vi "SNAKE AND LADDER 2 players final.vi"() -> ()   [LabVIEW 2018]
panel:
  out "dice 2":dbl(ring)
  out "dice 1":dbl(ring)
  out "WINNER":string
  out "Player 2":string
  out "PLAYER 2 LAST VALUE":dbl
  out "PLAYER 2":dbl
  out "PLAYER 2\nNEW VALUE":dbl
  out "NO.OF ROLLS":dbl
  out "PLAYER 1\nNEW VALUE":dbl
  out "PLAYER 1":dbl
  out "PLAYER 1 LAST VALUE":dbl
  out "Player 1":string
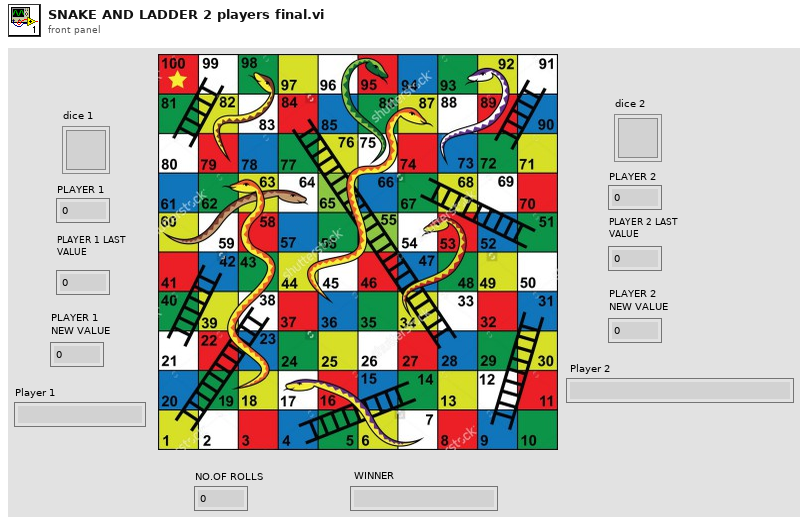
[diagram p1: front panel]
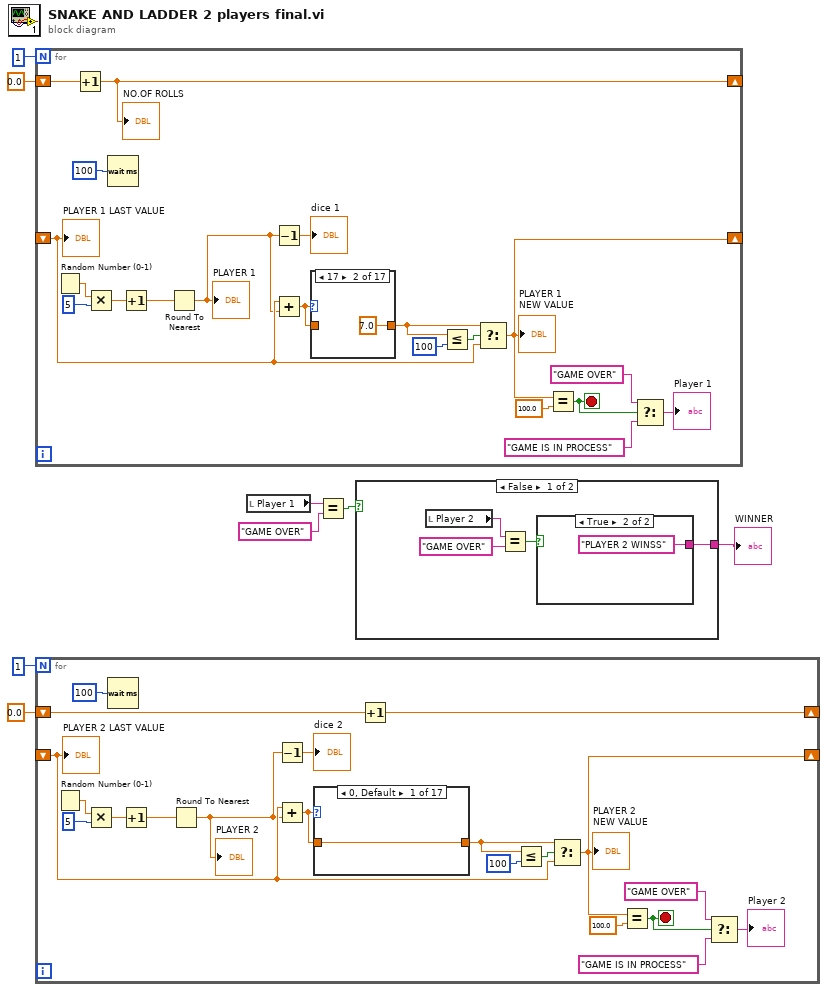
[diagram p0: block diagram]
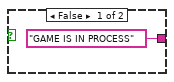
[diagram p2: hidden frame]
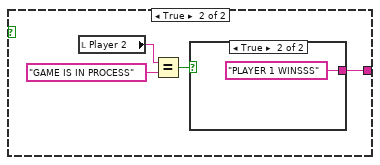
[diagram p3: hidden frame]
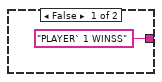
[diagram p4: hidden frame]
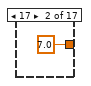
[diagram p5: hidden frame]
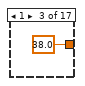
[diagram p6: hidden frame]
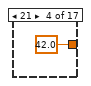
[diagram p7: hidden frame]
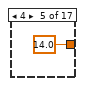
[diagram p8: hidden frame]
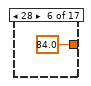
[diagram p9: hidden frame]
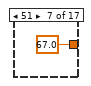
[diagram p10: hidden frame]
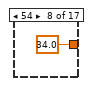
[diagram p11: hidden frame]
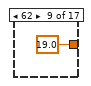
[diagram p12: hidden frame]
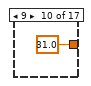
[diagram p13: hidden frame]
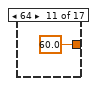
[diagram p14: hidden frame]
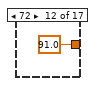
[diagram p15: hidden frame]
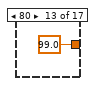
[diagram p16: hidden frame]
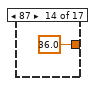
[diagram p17: hidden frame]
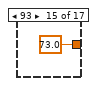
[diagram p18: hidden frame]
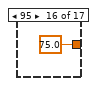
[diagram p19: hidden frame]
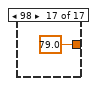
[diagram p20: hidden frame]
diagram:
  n1 = for {
    N: 1 -> [_]
    shift-right: [w18] -> _
    shift-left: _ -> [w14]
    shift-right: [w16] -> _
    shift-left: 0.0 -> [w17]
    stop <- w15 stop-if-true
    n2 = Random Number (0-1)() -> (number: 0 to 1=w28:dbl)
    n3 = Increment(x=w17) -> (x+1=w16:dbl)
    "NO.OF ROLLS" <- w16
    n4 = Multiply(x=w28, y=5) -> (x*y=w26:dbl)
    n5 = Wait (ms)(milliseconds to wait=u32 100 ("millisecond timer value")) -> ()  [unwired: 1 out]
    n6 = Increment(x=w26) -> (x+1=w25:dbl)
    n7 = Round To Nearest(number=w25) -> (nearest integer value=w10:dbl)
    "PLAYER 1" <- w10
    n8 = Decrement(x=w10) -> (x-1=→"dice 1":dbl)
    n9 = Add(x=w14, y=w10) -> (x+y=w24:dbl)
    n10 = case shown="17" w24 {
      tunnel: [w29 7.0 38.0 42.0 14.0 84.0 67.0 34.0 19.0 31.0 60.0 91.0 99.0 36.0 73.0 75.0 79.0] -> w13
      tunnel: w24 -> [w29 _ _ _ _ _ _ _ _ _ _ _ _ _ _ _ _]
      frame 0, Default {
      }
      frame 17 {
      }
      frame 1 {
      }
      frame 21 {
      }
      frame 4 {
      }
      frame 28 {
      }
      frame 51 {
      }
      frame 54 {
      }
      frame 62 {
      }
      frame 9 {
      }
      frame 64 {
      }
      frame 72 {
      }
      frame 80 {
      }
      frame 87 {
      }
      frame 93 {
      }
      frame 95 {
      }
      frame 98 {
      }
    }
    n11 = Less Or Equal?(x=w13, y=100) -> (x <= y?=w22:bool)
    n12 = Select(t=w13, s=w22, f=w14) -> (s? t:f=w18:dbl)
    "PLAYER 1\nNEW VALUE" <- w18
    n13 = Equal?(x=w18, y=100.0) -> (x = y?=w15:bool)
    n14 = Select(t="GAME OVER", s=w15, f="GAME IS IN PROCESS") -> (s? t:f=→"Player 1":string)
    "PLAYER 1 LAST VALUE" <- w14
  }
  n15 = for {
    N: 1 -> [_]
    shift-right: [w54] -> _
    shift-left: _ -> [w50]
    shift-right: [w52] -> _
    shift-left: 0.0 -> [w53]
    stop <- w51 stop-if-true
    n16 = Random Number (0-1)() -> (number: 0 to 1=w65:dbl)
    n17 = Multiply(x=w65, y=5) -> (x*y=w63:dbl)
    n18 = Wait (ms)(milliseconds to wait=u32 100 ("millisecond timer value")) -> ()  [unwired: 1 out]
    n19 = Increment(x=w63) -> (x+1=w62:dbl)
    n20 = Round To Nearest(number=w62) -> (nearest integer value=w46:dbl)
    "PLAYER 2" <- w46
    n21 = Decrement(x=w46) -> (x-1=→"dice 2":dbl)
    n22 = Add(x=w50, y=w46) -> (x+y=w61:dbl)
    n23 = case shown="0, Default" w61 {
      tunnel: [w66 7.0 38.0 42.0 14.0 84.0 67.0 34.0 19.0 31.0 60.0 91.0 99.0 36.0 73.0 75.0 79.0] -> w49
      tunnel: w61 -> [w66 _ _ _ _ _ _ _ _ _ _ _ _ _ _ _ _]
      frame 0, Default {
      }
      frame 17 {
      }
      frame 1 {
      }
      frame 21 {
      }
      frame 4 {
      }
      frame 28 {
      }
      frame 51 {
      }
      frame 54 {
      }
      frame 62 {
      }
      frame 9 {
      }
      frame 64 {
      }
      frame 72 {
      }
      frame 80 {
      }
      frame 87 {
      }
      frame 93 {
      }
      frame 95 {
      }
      frame 98 {
      }
    }
    n24 = Increment(x=w53) -> (x+1=w52:dbl)
    n25 = Less Or Equal?(x=w49, y=100) -> (x <= y?=w59:bool)
    n26 = Select(t=w49, s=w59, f=w50) -> (s? t:f=w54:dbl)
    "PLAYER 2\nNEW VALUE" <- w54
    n27 = Equal?(x=w54, y=100.0) -> (x = y?=w51:bool)
    n28 = Select(t="GAME OVER", s=w51, f="GAME IS IN PROCESS") -> (s? t:f=→"Player 2":string)
    "PLAYER 2 LAST VALUE" <- w50
  }
  n29 = local read "Player 1"() -> (w5:string)
  n30 = Equal?(x=w5, y="GAME OVER") -> (x = y?=w6:bool)
  n31 = case shown="False" w6 {
    tunnel: [w83 w89] -> w3
    frame False {
      n32 = local read "Player 2"() -> (w85:string)
      n33 = Equal?(x=w85, y="GAME OVER") -> (x = y?=w86:bool)
      n34 = case shown="True" w86 {
        tunnel: ["GAME IS IN PROCESS" "PLAYER 2 WINSS"] -> w83
        frame False {
        }
        frame True {
        }
      }
    }
    frame True {
      n35 = local read "Player 2"() -> (w92:string)
      n36 = Equal?(x=w92, y="GAME IS IN PROCESS") -> (x = y?=w90:bool)
      n37 = case shown="True" w90 {
        tunnel: ["PLAYER` 1 WINSS" "PLAYER 1 WINSSS" ("String 3")] -> w89
        frame False {
        }
        frame True {
        }
      }
    }
  }
  "WINNER" <- w3
